vi "instr_reportError.vi"(8 "error in (no error)":errorcluster, 10 "errorMsg":string, 11 "return type":i32) -> (0 "error out":errorcluster)   [LabVIEW 2019, in "Instrument.lvclass"]
uses:
  Instrument.lvclass
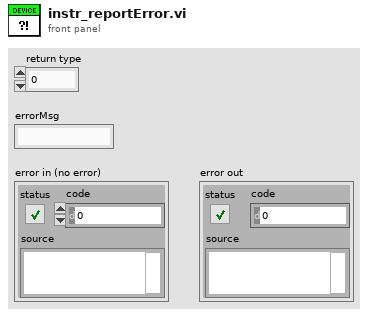
[diagram p1: front panel]
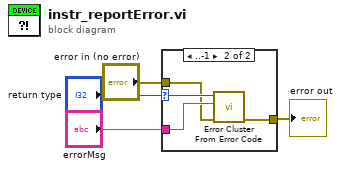
[diagram p0: block diagram]
diagram:
  n1 = case shown="..-1" "return type" {
    selector: "return type" -> [_ w9]
    tunnel: "errorMsg" -> [_ w8]
    tunnel: "error in (no error)" -> [w5 w7]
    tunnel: [w5 w6] -> w4
    frame 0, Default {
    }
    frame ..-1 {
      n2 = call <vilib>:"Error Cluster From Error Code.vi"("error in (no error)"=w7, "error message (\"\")"=w8, "error code (0)"=w9) -> ("error out"=w6:errorcluster)  [unwired: 6 in]
    }
  }
  "error out" <- w4
